vi "Get PDO Mappable Entries.vi"(8 "error in":errorcluster, 11 "Electronic Datasheet in":refnum<class "Electronic Datasheet.lvclass">) -> (0 "error out":errorcluster, 2 "PDO Mappable Entries":refnum<class "OD Entry.lvclass">[](array[class]), 3 "Electronic Datasheet out":refnum<class "Electronic Datasheet.lvclass">)   [LabVIEW 2024, in "Electronic Datasheet.lvlib" / "Electronic Datasheet.lvclass"]
uses:
  Electronic Datasheet.lvclass
  Core/OD Entry/OD Entry.lvclass
  Core/PDO Mapping Type.ctl
  Core/OD Sub-Entry/OD Sub-Entry.lvclass
  D:/git/EDS-File-Viewer/Core/OD Entry/OD Entry.lvclass
  Core/Electronic Datasheet.lvlib
  Core/Sorted Object Dictionary/Sorted Object Dictionary.lvclass
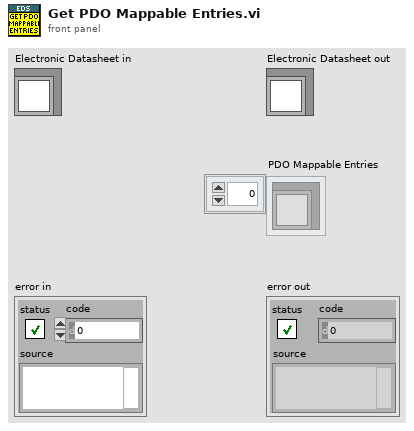
[diagram p1: front panel]
types:
  T1 = typedef "Electronic Datasheet.lvlib/PDO Mapping Type.ctl" = enum8{"NO", "OPTIONAL", "RPDO", "TPDO"}
  T2 = typedef "Electronic Datasheet.lvlib/Electronic Datasheet.lvclass/ObjectAttributes.ctl" = cluster{"EDS File Path":path, "Object Dict":refnum<class "Dictionary.lvclass">, "Sorted Object Dict":refnum<class "Sorted Object Dictionary.lvclass">, "Device Info":refnum<class "Device Info.lvclass">, "File Info":refnum<class "File Info.lvclass">}
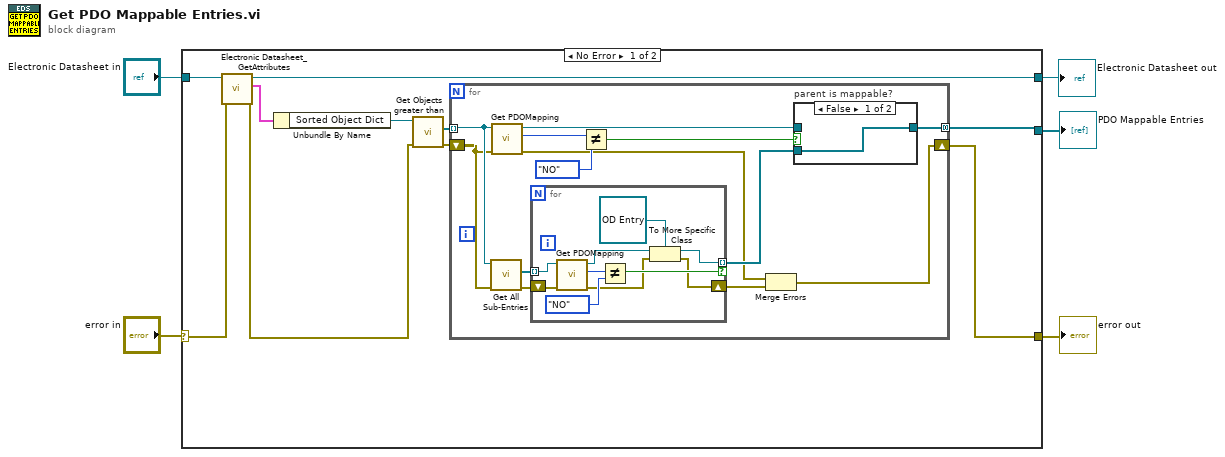
[diagram p0: block diagram]
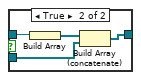
[diagram p2: hidden frame]
diagram:
  n1 = case shown="No Error" "error in" {
    selector: "error in" -> [w15 w45]
    tunnel: [w6 w45] -> w4
    tunnel: [w13 w44] -> w2
    tunnel: "Electronic Datasheet in" -> [w14 w44]
    tunnel: [w11 _] -> w1
    frame No Error {
      n2 = call "Electronic Datasheet_GetAttributes.vi"("Error In"=w15, "reference in"=w14) -> ("Error Out"=w12:errorcluster, "Data"=w7:T2, "reference out"=w13:refnum<class "Electronic Datasheet.lvclass">)  [unwired: 6 in, 1 out]
      n3 = Unbundle By Name(w7) -> ("Sorted Object Dict"=w10:refnum<class "Sorted Object Dictionary.lvclass">)
      n4 = call "Get Objects greater than.vi"("error in"=w12, "Sorted Object Dictionary in"=w10) -> ("error out"=w8:errorcluster, "Entries"=w9:refnum<class "OD Entry.lvclass">[])  [unwired: 7 in, 1 out]
      n5 = for {
        tunnel: w9 -> [w26] mode=indexing
        tunnel: [w19] -> w11 mode=concatenating
        shift-right: [w16] -> w6
        shift-left: w8 -> [w25]
        n6 = call "Get All Sub-Entries.vi"("Error In"=w25, "reference in"=w26) -> ("Error Out"=w24:errorcluster, "Sub-Entries"=w23:refnum<class "OD Sub-Entry.lvclass">[])  [unwired: 6 in, 2 out]
        n7 = call "Get PDOMapping.vi"("Error In"=w25, "reference in"=w26) -> ("Error Out"=w18:errorcluster, "PDOMapping"=w28:T1, "reference out"=w22:refnum<class "OD Entry.lvclass">)  [unwired: 7 in]
        n8 = for {
          tunnel: w23 -> [w42] mode=indexing
          tunnel: [w37] -> w20 mode=indexing if=w38
          shift-right: [w34] -> w17
          shift-left: w24 -> [w43]
          n9 = call "Get PDOMapping.vi"("Error In"=w43, "reference in"=w42) -> ("Error Out"=w35:errorcluster, "PDOMapping"=w41:T1, "reference out"=w39:refnum<class "OD Sub-Entry.lvclass">)  [unwired: 7 in]
          n10 = Not Equal?(x=w41, y=PDO_Mapping_Type."NO") -> (x != y?=w38:bool)
          n11 = To More Specific Class(target class=refnum<class "OD Entry.lvclass"> refnum ("Electronic Datasheet.lvlib:OD Entry"), reference=w39, error in=w35) -> (specific class reference=w37:refnum<class "OD Entry.lvclass">, error out=w34:errorcluster)
        }
        n12 = Not Equal?(x=w28, y=PDO_Mapping_Type."NO") -> (x != y?=w21:bool)
        n13 = Merge Errors(w18, w17) -> (w16:errorcluster)
        n14 = case "parent is mappable?" shown="False" w21 {
          tunnel: w22 -> [_ w33]
          tunnel: w20 -> [w29 w31]
          tunnel: [w29 w30] -> w19
          frame False {
          }
          frame True {
            n15 = Build Array(w33) -> (w32:refnum<class "OD Entry.lvclass">[])
            n16 = Build Array (concatenate)(w32, w31) -> (w30:refnum<class "OD Entry.lvclass">[])
          }
        }
      }
    }
    frame Error {
    }
  }
  "error out" <- w4
  "Electronic Datasheet out" <- w2
  "PDO Mappable Entries" <- w1
